vi "Get Measurements.vi"(8 "error in (no error)":errorcluster, 9 "High Speed":bool, 10 "HPS17K Refs":refnum<class "HPS-17000.lvclass">[](array[class]), 11 "Stream Queue":refnum<queue>) -> (0 "error out":errorcluster, 3 "Measurements":T1[](array[typedef]))   [LabVIEW 2023]
uses:
  <vilib>/HPS-17000/MStream_grpc_CyclerMeasurement.ctl
  <instrlib>/HPS-17000/HPS-17000.lvclass
  <instrlib>/HPS-17000/Internal/Read Measurement Multi.vi
  <vilib>/HPS-17000/NI_BC_client.lvlib
panel:
  in  "Cycler Selection":i16
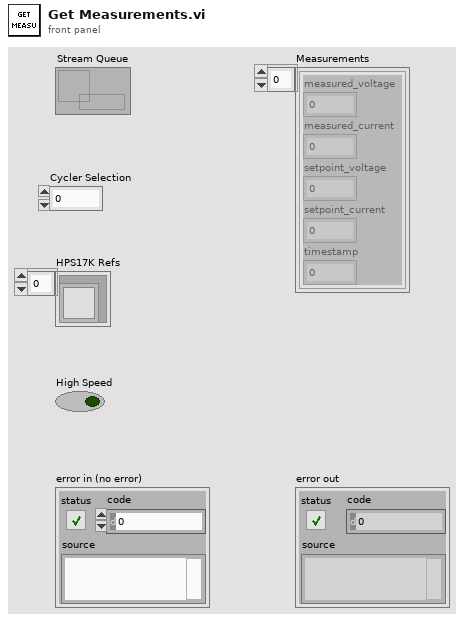
[diagram p1: front panel]
types:
  T1 = typedef "NI_BC_client.lvlib/MStream_grpc_CyclerMeasurement.ctl" = cluster{"measured_voltage":sgl, "measured_current":sgl, "setpoint_voltage":sgl, "setpoint_current":sgl, "timestamp":i64}
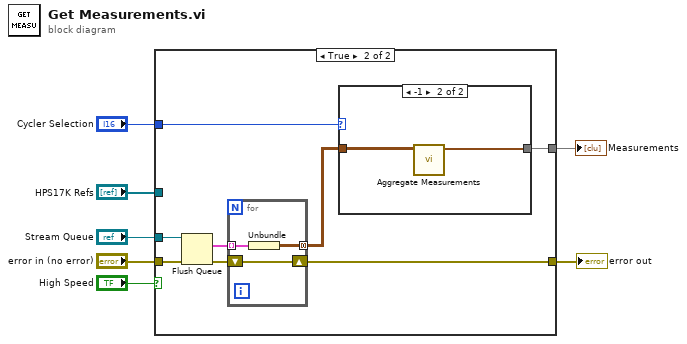
[diagram p0: block diagram]
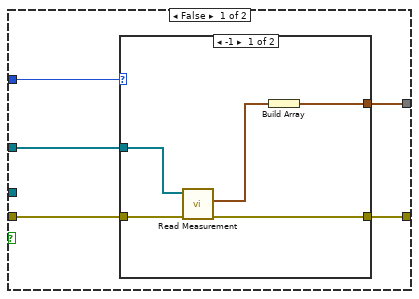
[diagram p2: hidden frame]
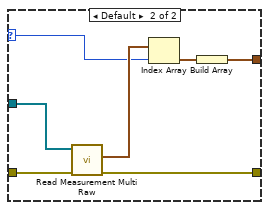
[diagram p3: hidden frame]
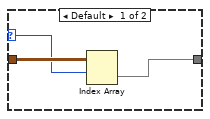
[diagram p4: hidden frame]
diagram:
  n1 = case shown="True" "High Speed" {
    tunnel: "HPS17K Refs" -> [w10 _]
    tunnel: "error in (no error)" -> [w12 w32]
    tunnel: [w11 w28] -> w5
    tunnel: "Stream Queue" -> [_ w31]
    tunnel: "Cycler Selection" -> [w9 w27]
    tunnel: [w8 w26] -> w1
    frame False {
      n2 = case shown="-1" w9 {
        selector: w9 -> [_ w20]
        tunnel: w12 -> [w17 w24]
        tunnel: [w15 w23] -> w11
        tunnel: w10 -> [w16 w22]
        tunnel: [w13 w18] -> w8
        frame -1 {
          n3 = call-poly <instrlib>:"Read Measurement.vi"("error in"=w17, "cycler refs in"=w16) -> ("error out"=w15:errorcluster, "aggregated cycler measurements"=w14:T1)  [unwired: 7 in, 1 out]
          n4 = Build Array(w14) -> (w13:T1[])
        }
        frame Default {
          n5 = call <instrlib>:"Read Measurement Multi Raw.vi"("error in"=w24, "cycler refs in"=w22) -> ("error out"=w23:errorcluster, "cycler measurements"=w21:T1[])  [unwired: 7 in, 1 out]
          n6 = Index Array(array=w21, index=w20) -> (element=w19:T1)
          n7 = Build Array(w19) -> (w18:T1[])
        }
      }
    }
    frame True {
      n8 = Flush Queue(queue=w31, error in (no error)=w32) -> (remaining elements=w30:cluster{T1[][]}[], error out=w29:errorcluster)  [unwired: 1 out]
      n9 = for {
        tunnel: w30 -> [w39] mode=indexing
        shift-right: [w40] -> w28
        shift-left: w29 -> [w40]
        tunnel: [w38] -> w25 mode=concatenating
        n10 = Unbundle(w39) -> (w38:T1[][])
      }
      n11 = case shown="-1" w27 {
        selector: w27 -> [w34 _]
        tunnel: w25 -> [w35 w37]
        tunnel: [w33 w36] -> w26
        frame Default {
          n12 = Index Array(array=w35, index (row)=w34) -> (element=w33:T1[])  [unwired: 1 in]
        }
        frame -1 {
          n13 = call <instrlib>:"Aggregate Measurements.vi"("cycler measurements"=w37) -> ("cycler measurements"=w36:T1[])  [unwired: 10 in]
        }
      }
    }
  }
  "Measurements" <- w1
  "error out" <- w5
